vi "ZDataVIS_Select_Intensity.vi"(5 "Z":T1(ring), 6 "Y":T1(ring), 7 "X":T1(ring), 8 "error in (no error)":errorcluster, 9 "Slow Index (Row)":dbl, 10 "Slowest Index (Page)":i32, 11 "Big Ol Array IN":T2(array[cluster])) -> (0 "error out":errorcluster, 3 "Intensity Info OUT":cluster{dbl[], dbl[]}[](array[cluster]))   [LabVIEW 2016]
panel:
  out "2term Intensity":dbl[][](graph)
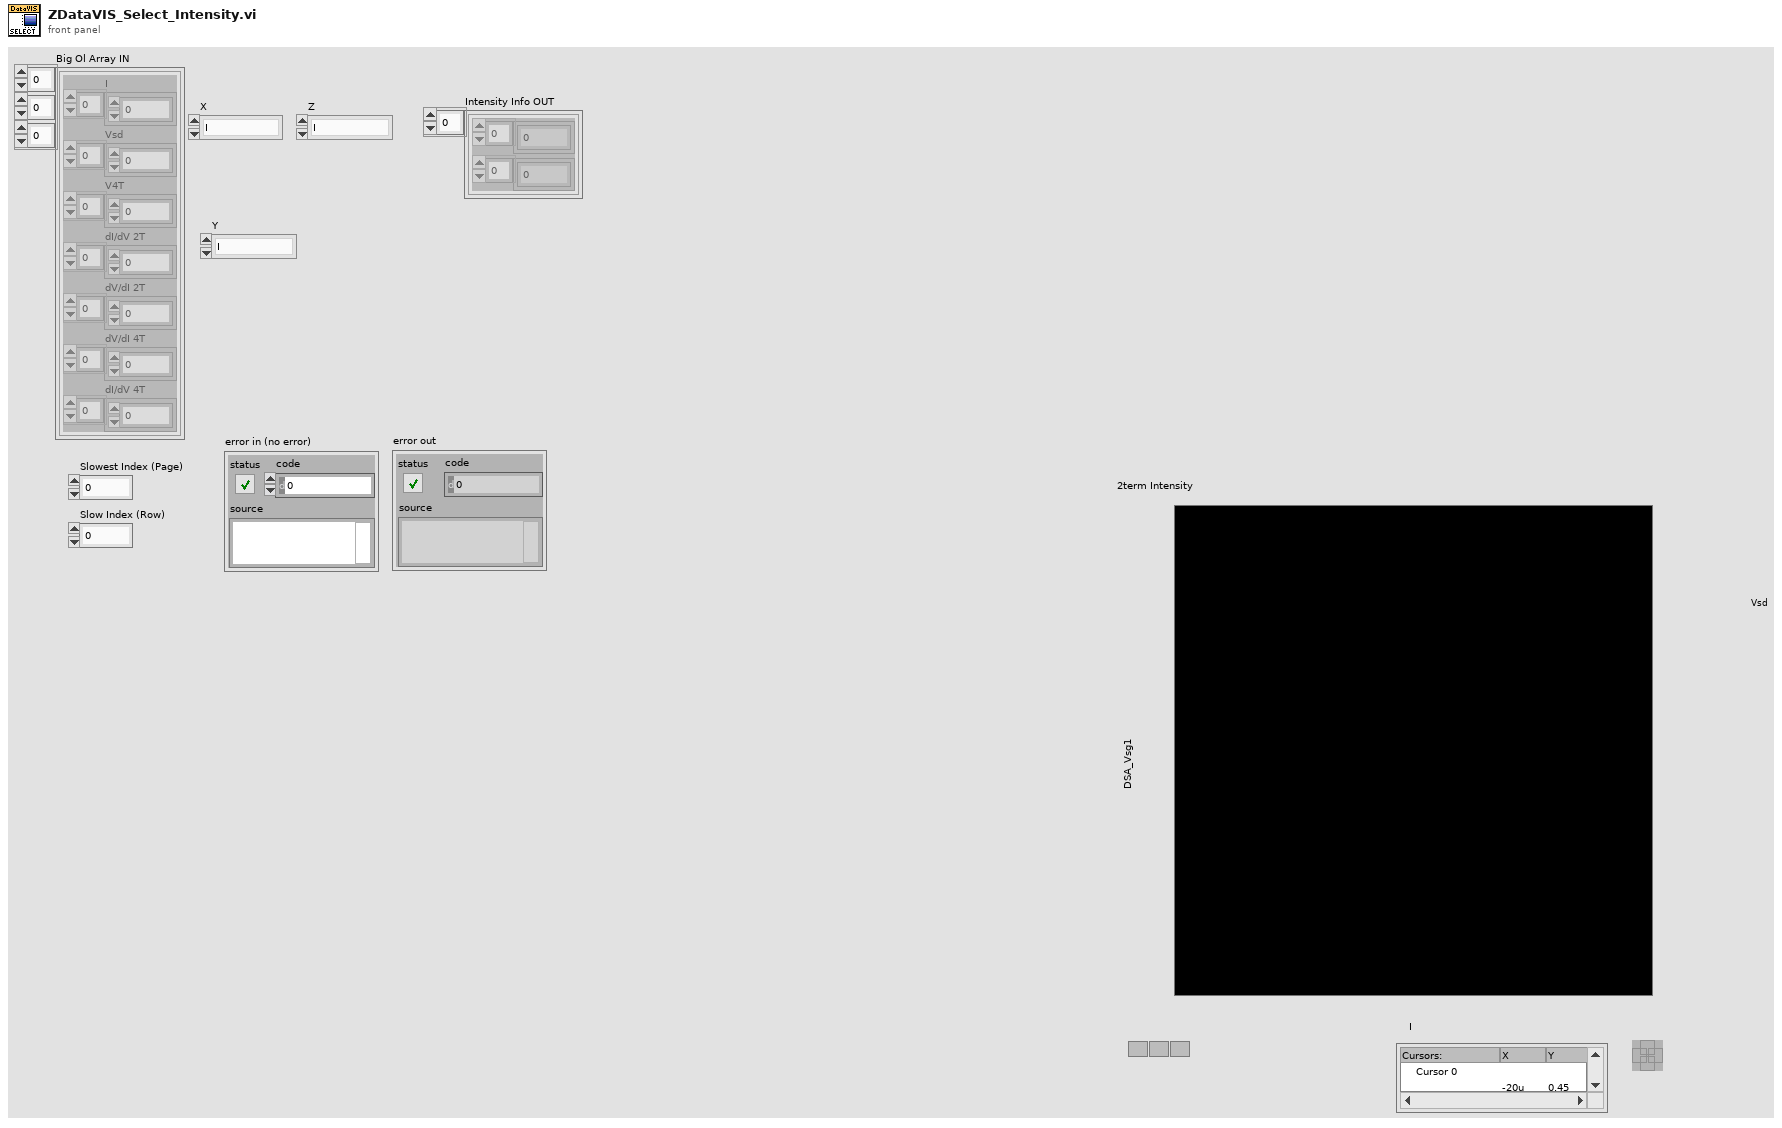
[diagram p1: front panel]
types:
  T1 = enum16{"I", "Vsd", "V4T", "dI/dV 2T", "dV/dI 2T", "dV/dI 4T", "dI/dV 4T"}
  T2 = cluster{"I":dbl[], "Vsd":dbl[], "V4T":dbl[], "dI/dV 2T":dbl[], "dV/dI 2T":dbl[], "dV/dI 4T":dbl[], "dI/dV 4T":dbl[]}[][][]
  T3 = cluster{"I":dbl[], "Vsd":dbl[], "V4T":dbl[], "dI/dV 2T":dbl[], "dV/dI 2T":dbl[], "dV/dI 4T":dbl[], "dI/dV 4T":dbl[]}[]
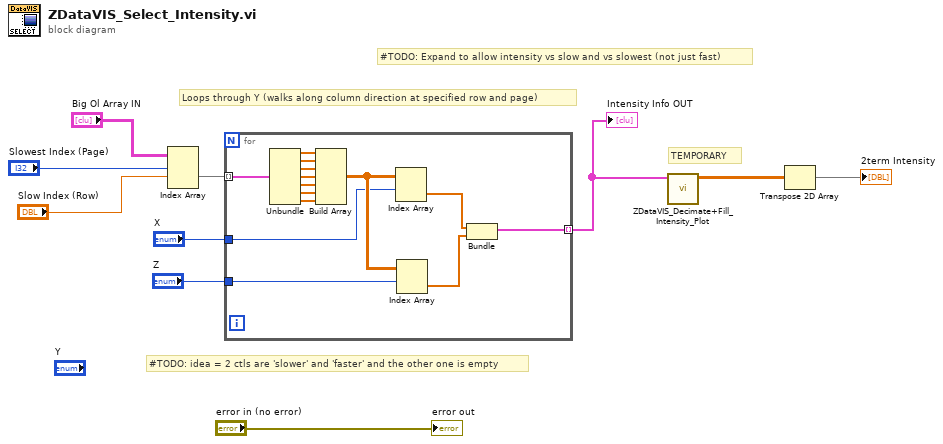
[diagram p0: block diagram]
diagram:
  # "TEMPORARY"
  # "Loops through Y (walks along column direction at specified row and page)"
  # "#TODO: idea = 2 ctls are 'slower' and 'faster' and the other one is empty"
  # "#TODO: Expand to allow intensity vs slow and vs slowest (not just fast)"
  n1 = Index Array(array="Big Ol Array IN", index (dim 0)="Slowest Index (Page)", index (dim 1)="Slow Index (Row)") -> (element=w9:T3)  [unwired: 1 in]
  n2 = for {
    tunnel: w9 -> [w17] mode=indexing
    tunnel: [w13] -> w2 mode=indexing
    tunnel: "X" -> [w12]
    tunnel: "Z" -> [w11]
    n3 = Unbundle(w17) -> ("I"=w24:dbl[], "Vsd"=w23:dbl[], "V4T"=w22:dbl[], "dI/dV 2T"=w21:dbl[], "dV/dI 2T"=w20:dbl[], "dV/dI 4T"=w19:dbl[], "dI/dV 4T"=w18:dbl[])
    n4 = Build Array(w24, w23, w22, w21, w20, w19, w18) -> (w16:dbl[][])
    n5 = Index Array(array=w16, index (row)=w12) -> (element=w14:dbl[])  [unwired: 1 in]
    n6 = Index Array(array=w16, index (row)=w11) -> (element=w15:dbl[])  [unwired: 1 in]
    n7 = Bundle(w14, w15) -> (w13:cluster{dbl[], dbl[]})  [unwired: 1 in]
  }
  "Intensity Info OUT" <- w2
  n8 = call "ZDataVIS_Decimate+Fill_Intensity_Plot.vi"("X and Y Arrays to decimate"=w2) -> ("Arr of Y arrays (intensity info)"=w4:dbl[][])  [unwired: 8 in, 2 out]
  n9 = Transpose 2D Array(2D array=w4) -> (transposed array=→"2term Intensity":dbl[][])
  "error out" <- "error in (no error)"
